vi "Analog Input.vi"() -> ()   [LabVIEW 2012]
uses:
  <vilib>/DAQmx/read.llb/DAQmx Read (Analog DBL 1Chan 1Samp).vi
  <vilib>/DAQmx/create/channels.llb/DAQmx Create Channel (AI-Voltage-Basic).vi
  <vilib>/DAQmx/miscellaneous.llb/DAQmx Fill In Error Info.vi
panel:
  out "Voltage Meter":dbl(knob) scale=0.0..5.0
  in  "physical \nchannels":tag
  in  "?":bool
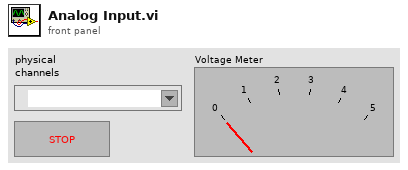
[diagram p1: front panel]
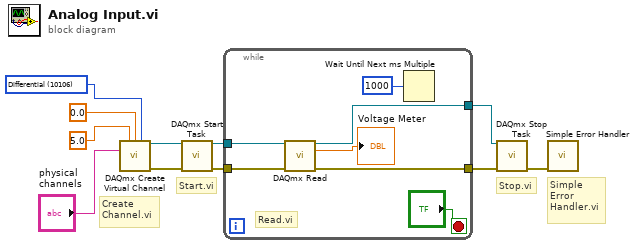
[diagram p0: block diagram]
diagram:
  w3 = 10106 items=["default"=-1, "RSE"=10083, "NRSE"=10078, "Differential"=10106, "Pseudodifferential"=12529] ("input terminal configuration")
  # "Simple\nError\nHandler.vi"
  # "Stop.vi"
  # "Start.vi"
  # "Create\nChannel.vi"
  n1 = call-poly <vilib>:"DAQmx Create Virtual Channel.vi"("maximum value"=5.0, "minimum value"=0.0, "input terminal configuration"=w3, "physical channels"="physical \nchannels") -> ("task out"=w10:refnum<k21>, "error out"=w9:errorcluster)  [unwired: 10 in]
  n2 = call <vilib>:"DAQmx Start Task.vi"("task/channels in"=w10, "error in"=w9) -> ("task out"=w7:refnum<k21>, "error out"=w8:errorcluster)  [unwired: 12 in]
  n3 = while {
    tunnel: w8 -> [w16]
    tunnel: w7 -> [w17]
    tunnel: [w15] -> w6
    tunnel: [w14] -> w4
    stop <- "?" stop-if-true
    # "Read.vi"
    n4 = call-poly <vilib>:"DAQmx Read.vi"("task/channels in"=w17, "error in"=w16) -> ("task out"=w14:refnum<k21>, "data"=→"Voltage Meter":dbl, "error out"=w15:errorcluster)  [unwired: 11 in]
    n5 = Wait Until Next ms Multiple(millisecond multiple=u32 1000) -> ()  [unwired: 1 out]
  }
  n6 = call <vilib>:"DAQmx Stop Task.vi"("task/channels in"=w4, "error in"=w6) -> ("error out"=w5:errorcluster)  [unwired: 12 in, 1 out]
  n7 = call <vilib>:"Simple Error Handler.vi"("error in (no error)"=w5) -> ()  [unwired: 4 in, 5 out]
